vi "Write log file.vi"(8 "error in (no error)":errorcluster) -> (0 "error out":errorcluster)   [LabVIEW 2016]
uses:
  Typedef/Remote Control Cluster.ctl
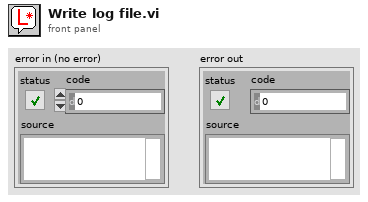
[diagram p1: front panel]
types:
  T1 = typedef "Remote Control Cluster.ctl" = cluster{"Pot1":u16, "Pot2":u16, "Pot3":u16, "Pot4":u16, "Switch1":cluster{"L":bool, "H":bool}, "Switch2":cluster{"L":bool, "H":bool}, "Switch3":cluster{"L":bool, "H":bool}}
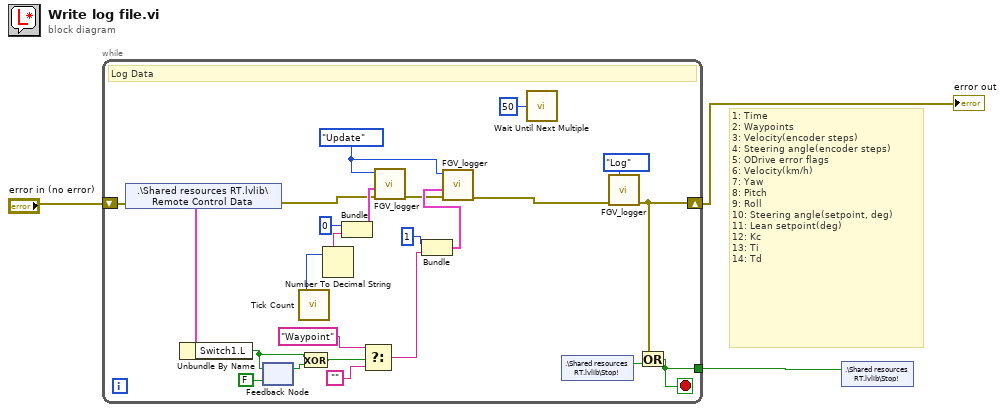
[diagram p0: block diagram]
diagram:
  # "1: Time\n2: Waypoints\n3: Velocity(encoder steps)\n4: Steering angle(encoder steps)\n5: ODrive error flags\n6: Velocity(km/h)\n7: Yaw\n8: Pitch\n9: Roll\n10: Steering angle(setpoint, deg)\n11: Lean setpoint(deg)\n12: Kc\n13: Ti\n14: Td"
  n1 = while {
    tunnel: [w26] -> w1
    shift-right: [w20] -> w3
    shift-left: "error in (no error)" -> [w17]
    stop <- w26 stop-if-true
    w19 = enum16{"Update", "Log", "Init"}."Update" ("Command")
    # "Log Data"
    n2 = shared-variable ".\\Shared resources RT.lvlib\\Remote Control Data"(error in=w17) -> (w15:T1, error out=w16:errorcluster)
    n3 = Unbundle By Name(w15) -> ("Switch1.L"=w4:bool)
    n4 = feedback-in #1(w4) -> ()
    n5 = feedback #1(FALSE ("L")) -> (w6:bool)
    n6 = call "Tick Count"() -> ("Tick Count(mSec)"=w21:u32)
    n7 = Exclusive Or(1:w6, 2:w4) -> (0:w5:bool)
    n8 = Number To Decimal String(number=w21) -> (decimal integer string=w22:string)  [unwired: 1 in]
    n9 = Bundle(0, w22) -> (w24:cluster{i32, string})  [unwired: 1 in]
    n10 = Select(t="Waypoint", s=w5, f="") -> (s? t:f=w11:string)
    n11 = call "FGV_logger.vi"("error in"=w16, 9:w24, "Command"=w19) -> ("error out"=w9:errorcluster)  [unwired: 8 in]
    n12 = Bundle(1, "t"=w11) -> (w10:cluster{i32, "t":string})  [unwired: 1 in]
    n13 = call "FGV_logger.vi"("error in"=w9, 9:w10, "Command"=w19) -> ("error out"=w8:errorcluster)  [unwired: 8 in]
    n14 = call "Wait Until Next Multiple"("Count(mSec)"=u32 50) -> ()  [unwired: 1 out]
    n15 = shared-variable ".\\Shared resources RT.lvlib\\Stop!"() -> (w27:bool)  [unwired: 1 in, 1 out]
    n16 = call "FGV_logger.vi"("error in"=w8, "Command"=enum16{"Update", "Log", "Init"}."Log") -> ("error out"=w20:errorcluster)  [unwired: 9 in]
    n17 = Or(x=w20, y=w27) -> (x .or. y?=w26:bool)
  }
  "error out" <- w3
  n18 = shared-variable ".\\Shared resources RT.lvlib\\Stop!"(w1) -> ()  [unwired: 1 in, 1 out]
